vi "Periodic Tasks.vi"(8 "error in":errorcluster) -> ()   [LabVIEW 2017]
doc: "This VI runs in parallel to other tasks. It can contain as many user-defined periodic loops as you need. These can carry out PID or other sorts of timed response."
uses:
  <vilib>/Rock Robotics/WPI/Utilities/WPI_GetSetVariantRefNum.vi
  <vilib>/Rock Robotics/WPI/Ultrasonic/WPI_SonarMB1010AnalogRefNum Registry Get.vi
  Robot Global Data.vi
  <vilib>/Rock Robotics/WPI/Ultrasonic/WPI_SonarMB1010AnalogGetRange.vi
  <vilib>/Rock Robotics/Network Tables/NT Write Number.vi
  <vilib>/Rock Robotics/Network Tables/NT Write Numeric Array.vi
panel:
  out "Blinky":bool
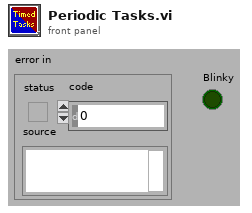
[diagram p1: front panel]
types:
  T1 = typedef "WPI_SonarMB1010AnalogDeviceRef.ctl" = cluster{"AIDeviceRef":T2, "Scaling factor (V/in)":dbl, "Average Bits":u8}
  T2 = typedef "WPI_AnalogChannelDevRef.ctl" = cluster{"DevStatus":errorcluster, "Analog Channel":T3}
  T3 = typedef "FPGA_AIChannel.ctl" = enum8{"AI 0", "AI 1", "AI 2", "AI 3", "AI MXP 0", "AI MXP 1", "AI MXP 2", "AI MXP 3", "Invalid"}
  T4 = typedef "WPI_GyroDevRef.ctl" = cluster{"DevStatus":errorcluster, "Analog Channel":T3, "Gain (VoltsPerDegree/Second)":dbl, "Gyro Type":enum16{"Analog", "XRS450"}, "Handle":i32, "SPI Bus":T5, "Device Found":bool, "Sample Rate":dbl, "Calibrate On Open":bool, "Offset":dbl}
  T5 = typedef "spi_bus.ctl" = enum16{"SPI On-Board, CS0", "SPI On-Board, CS1", "SPI On-Board, CS2", "SPI On-Board, CS3", "SPI MXP", "Invalid"}
  T6 = typedef "WPI_JoystickDevRef.ctl" = cluster{"Device":T7}
  T7 = typedef "WPI_JoystickDeviceEnum.ctl" = enum16{"USB 0", "USB 1", "USB 2", "USB 3", "USB 4", "USB 5"}
  T8 = typedef "WPI_DigitalInputDevRef.ctl" = cluster{"DevStatus":errorcluster, "DIO Channel":T9}
  T9 = typedef "FPGA_DIOChannel.ctl" = enum8{"DIO 0", "DIO 1", "DIO 2", "DIO 3", "DIO 4", "DIO 5", "DIO 6", "DIO 7", "DIO 8", "DIO 9", "DIO MXP 0", "DIO MXP 1", "DIO MXP 2", "DIO MXP 3", "DIO MXP 4", "DIO MXP 5", "DIO MXP 6", "DIO MXP 7", "DIO MXP 8", "DIO MXP 9", "DIO MXP 10", "DIO MXP 11", "DIO MXP 12", "DIO MXP 13", "DIO MXP 14", "DIO MXP 15", "SPI Port CS1", "SPI Port CS2", "SPI Port CS3", "SPI Port MISO", "SPI Port MOSI", "Invalid"}
  T10 = cluster{"GyroDevRef":T4, "JoystickDevRef":T6, "SonarMB1010AnalogDevRef":T1, "DigitalInputDevRef":T8}
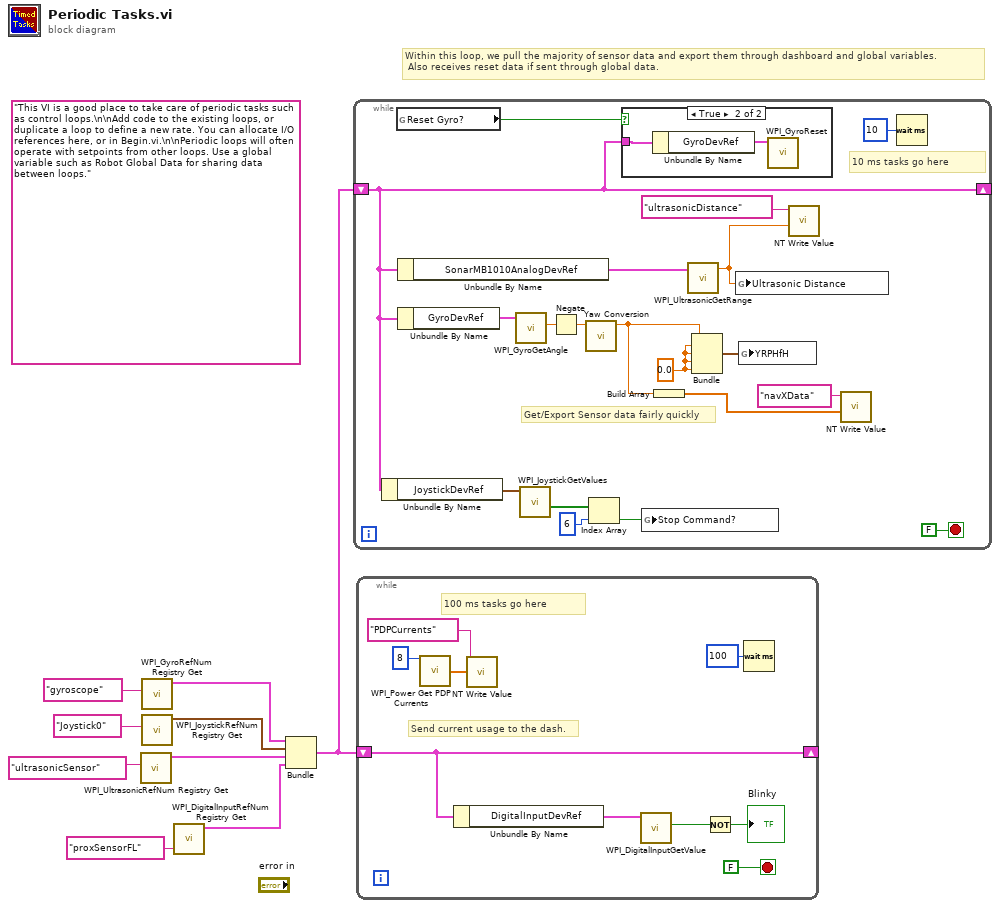
[diagram p0: block diagram]
diagram:
  (unwired) "This VI is a good place to take care of periodic tasks such as control loops.\n\nAdd code to the existing loops, or duplicate a loop to define a new rate. You can allocate I/O references here, or in Begin.vi.\n\nPeriodic loops will often operate with setpoints from other loops. Use a global variable such as Robot Global Data for sharing data between loops."
  # "Within this loop, we pull the majority of sensor data and export them through dashboard and global variables.\n Also receives reset data if sent through global data."
  n1 = call-poly <vilib>:"WPI_UltrasonicRefNum Registry Get.vi"("refnum name"="ultrasonicSensor") -> ("SonarMB1010AnalogDevRef"=w4:T1)  [unwired: 9 in, 1 out]
  n2 = call <vilib>:"WPI_GyroRefNum Registry Get.vi"("refnum name"="gyroscope") -> ("GyroDevRef"=w5:T4)  [unwired: 9 in, 1 out]
  n3 = call <vilib>:"WPI_JoystickRefNum Registry Get.vi"("refnum name"="Joystick0") -> ("JoystickDevRef"=w9:T6)  [unwired: 9 in, 1 out]
  n4 = call <vilib>:"WPI_DigitalInputRefNum Registry Get.vi"("refnum name"="proxSensorFL") -> ("DigitalInputDevRef"=w2:T8)  [unwired: 9 in, 1 out]
  n5 = Bundle("GyroDevRef"=w5, "JoystickDevRef"=w9, "SonarMB1010AnalogDevRef"=w4, "DigitalInputDevRef"=w2) -> (w7:T10)  [unwired: 1 out]
  n6 = while {
    shift-right: [w20] -> _
    shift-left: w7 -> [w20]
    stop <- FALSE stop-if-true
    w22 = 0.0
    # "Get/Export Sensor data fairly quickly"
    # "10 ms tasks go here"
    n7 = Unbundle By Name(w20) -> ("JoystickDevRef"=w19:T6)
    n8 = global read "Robot Global Data.vi" "Reset Gyro?"() -> (w21:bool)
    n9 = Unbundle By Name(w20) -> ("SonarMB1010AnalogDevRef"=w12:T1)
    n10 = Unbundle By Name(w20) -> ("GyroDevRef"=w25:T4)
    n11 = call <vilib>:"WPI_GyroGetAngle.vi"("GyroDevRef"=w25) -> ("Angle"=w13:dbl)  [unwired: 6 in, 4 out]
    n12 = call <vilib>:"WPI_JoystickGetValues.vi"("JoystickDevRef"=w19) -> ("Buttons"=w18:bool[])  [unwired: 6 in, 4 out]
    n13 = Negate(x=w13) -> (-x=w15:dbl)
    n14 = call "Yaw Conversion.vi"("Input"=w15) -> ("Output"=w14:dbl)  [unwired: 10 in]
    n15 = Index Array(array=w18, index=6) -> (element=w16:bool)
    n16 = case shown="True" w21 {
      tunnel: w20 -> [_ w30]
      frame False {
      }
      frame True {
        n17 = Unbundle By Name(w30) -> ("GyroDevRef"=w29:T4)
        n18 = call <vilib>:"WPI_GyroReset.vi"("GyroDevRef"=w29) -> ()  [unwired: 9 in, 2 out]
      }
    }
    n19 = global write "Robot Global Data.vi" "Stop Command?"(w16) -> ()
    n20 = Build Array(w14) -> (w24:dbl[])
    n21 = call-poly <vilib>:"WPI_UltrasonicGetRange.vi"("SonarMB1010AnalogDevRef"=w12) -> ("Distance"=w11:dbl)  [unwired: 8 in, 2 out]
    n22 = Bundle("Output"=w14, w22, w22, w22, w22) -> (w23:cluster{"Output":dbl, dbl, dbl, dbl, dbl})  [unwired: 1 in]
    n23 = global write "Robot Global Data.vi" "Ultrasonic Distance"(w11) -> ()
    n24 = global write "Robot Global Data.vi" "YRPHfH"(w23) -> ()
    n25 = call-poly <vilib>:"NT Write Value.vi"("Numeric"=w11, "Name"="ultrasonicDistance") -> ()  [unwired: 9 in, 1 out]
    n26 = call-poly <vilib>:"NT Write Value.vi"("Numeric Array"=w24, "Name"="navXData") -> ()  [unwired: 9 in, 1 out]
    n27 = Wait (ms)(milliseconds to wait=u32 10) -> ()  [unwired: 1 out]
  }
  n28 = while {
    shift-right: [w33] -> _
    shift-left: w7 -> [w33]
    stop <- FALSE stop-if-true
    # "Send current usage to the dash."
    # "100 ms tasks go here"
    n29 = call <vilib>:"WPI_Power Get PDP Currents.vi"("Power Distribution Panel (0)"=u8 8) -> ("all currents (A)"=w37:dbl[])  [unwired: 12 in, 2 out]
    n30 = Unbundle By Name(w33) -> ("DigitalInputDevRef"=w34:T8)
    n31 = call-poly <vilib>:"NT Write Value.vi"("Numeric Array"=w37, "Name"="PDPCurrents") -> ()  [unwired: 9 in, 1 out]
    n32 = call <vilib>:"WPI_DigitalInputGetValue.vi"("DigitalInputDevRef"=w34) -> ("Value"=w32:bool)  [unwired: 8 in, 2 out]
    n33 = Not(x=w32) -> (.not. x?=→"Blinky":bool)
    n34 = Wait (ms)(milliseconds to wait=u32 100) -> ()  [unwired: 1 out]
  }
